vi "Get Tuner Type.vi"(8 "error in (no error)":errorcluster, 11 "RTL-SDR in":refnum<class "RTL-SDR.lvclass">) -> (0 "error out":errorcluster, 1 "function return":i32, 2 "Tuner Type":T1, 3 "RTL-SDR out":refnum<class "RTL-SDR.lvclass">)   [LabVIEW 2015, in "RTL-SDR.lvclass"]
doc: "Created IvanLis by LabVIEW Portal\nProfile: http://labviewportal.org/memberlist.php?mode=viewprofile&u=987\neMail: IvanLisanov@gMail.com\nTelegram: https://t.me/IvanLis"
uses:
  RTL-SDR.lvclass
  TypeDef/Tuner Type.ctl
  RTL-SDR.lvclass/RTL-SDR.ctl
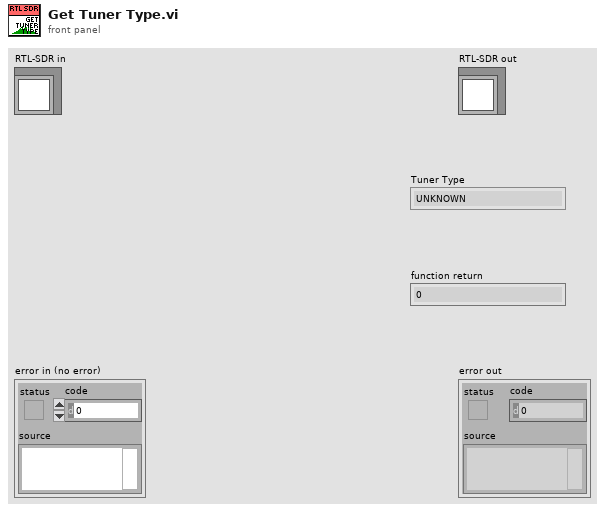
[diagram p1: front panel]
types:
  T1 = typedef "RTL-SDR.lvclass/Tuner Type.ctl" = enum16{"UNKNOWN", "E4000", "FC0012", "FC0013", "FC2580", "R820T", "R828D"}
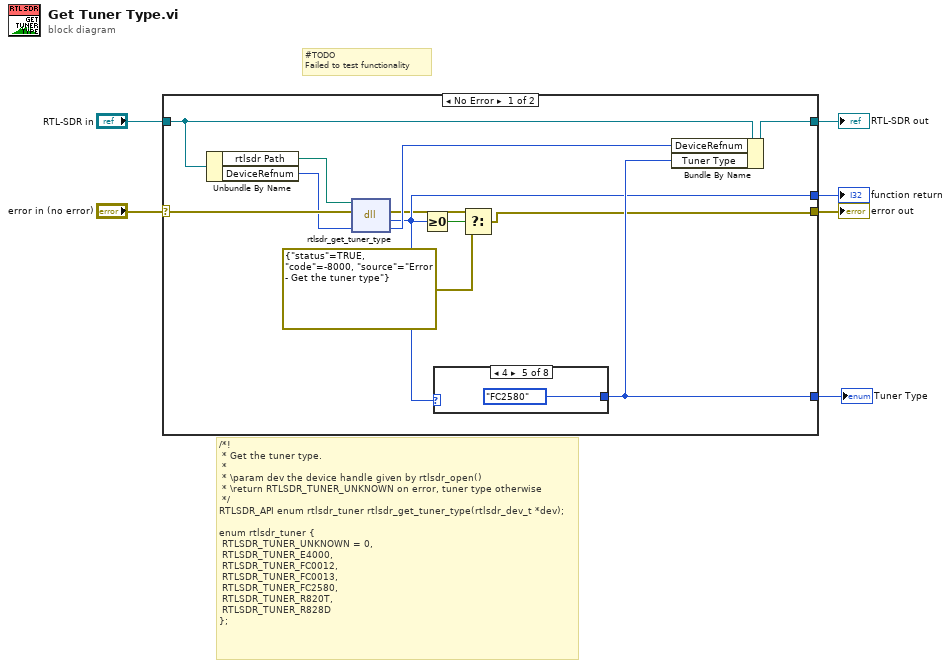
[diagram p0: block diagram]
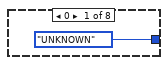
[diagram p2: hidden frame]
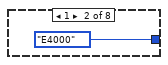
[diagram p3: hidden frame]
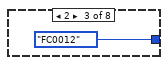
[diagram p4: hidden frame]
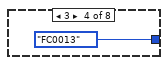
[diagram p5: hidden frame]
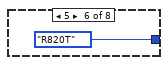
[diagram p6: hidden frame]
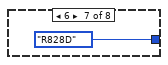
[diagram p7: hidden frame]
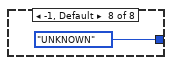
[diagram p8: hidden frame]
diagram:
  # "#TODO\nFailed to test functionality"
  # "/*!\n * Get the tuner type.\n *\n * \\param dev the device handle given by rtlsdr_open()\n * \\return RTLSDR_TUNER_UNKNOWN on error, tuner type otherwise\n */\nRTLSDR_API enum rtlsdr_tuner rtlsdr_get_tuner_type(rtlsdr_dev_t *dev);\n\nenum rtlsdr_tuner {\n\tRTLSDR_TUNER_UNKNOWN = 0,\n\tRTLSDR_TUNER_E4000,\n\tRTLSDR_TUNER_FC0012,\n\tRTLSDR_TUNER_FC0013,\n\tRTLSDR_TUNER_FC2580,\n\tRTLSDR_TUNER_R820T,\n\tRTLSDR_TUNER_R828D\n};"
  n1 = case shown="No Error" "error in (no error)" {
    selector: "error in (no error)" -> [w18 w28]
    tunnel: [w7 w28] -> w5
    tunnel: [w14 w27] -> w3
    tunnel: "RTL-SDR in" -> [w17 w27]
    tunnel: [w9 _] -> w2
    tunnel: [w12 _] -> w1
    frame No Error {
      n2 = Unbundle By Name(w17) -> ("rtlsdr Path"=w16:path, "DeviceRefnum"=w15:u64)
      n3 = dll-call lib="C:/Users/Ivan/Desktop/RTL-SDR Class_lv2015/Project (RTL-SDR)/RTL-SDR Class/dll/rtlsdr.dll" fn="rtlsdr_get_tuner_type"(path in=w16, error in=w18, "DeviceRefnum"=w15) -> (error out=w8:errorcluster, "return type"=w9:i32, "DeviceRefnum"=w13:u64)  [unwired: 1 in, 1 out]
      n4 = Greater Or Equal To 0?(x=w9) -> (x >= 0?=w11:bool)
      n5 = case shown="4" w9 {
        tunnel: [Tuner_Type."UNKNOWN" Tuner_Type."E4000" Tuner_Type."FC0012" Tuner_Type."FC0013" Tuner_Type."FC2580" Tuner_Type."R820T" Tuner_Type."R828D" Tuner_Type."UNKNOWN"] -> w12
        frame 0 {
        }
        frame 1 {
        }
        frame 2 {
        }
        frame 3 {
        }
        frame 4 {
        }
        frame 5 {
        }
        frame 6 {
        }
        frame -1, Default {
        }
      }
      n6 = Select(t=w8, s=w11, f=errorcluster {"status"=TRUE, "code"=-8000, "source"="Error - Get the tuner type"} ("error out")) -> (s? t:f=w7:errorcluster)
      n7 = Bundle By Name(cluster=w17, "DeviceRefnum"=w13, "Tuner Type"=w12) -> (w14:refnum<class "RTL-SDR.lvclass">)
    }
    frame Error {
    }
  }
  "error out" <- w5
  "RTL-SDR out" <- w3
  "Tuner Type" <- w1
  "function return" <- w2
